vi "Read Status.vi"(8 "error in (no error)":errorcluster, 11 "LFCSimShutt in":refnum<class "LFCSimShutt.lvclass">) -> (0 "error out":errorcluster, 2 "Status":bool, 3 "LFCSimShutt out":refnum<class "LFCSimShutt.lvclass">)   [LabVIEW 2016, in "LFCSimShutt.lvclass"]
uses:
  LFCSimShutt.lvclass
  Shutter.lvclass
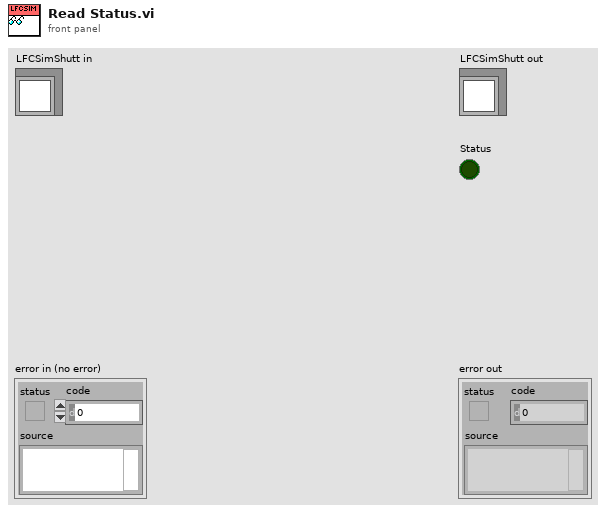
[diagram p1: front panel]
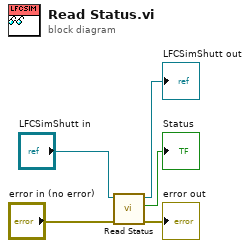
[diagram p0: block diagram]
diagram:
  n1 = call-parent "Read Status.vi"("error in (no error)"="error in (no error)", "Shutter in"="LFCSimShutt in") -> ("error out"=→"error out":errorcluster, "Status"=→"Status":bool, "Shutter out"=→"LFCSimShutt out":refnum<class "LFCSimShutt.lvclass">)  [unwired: 7 in]
